vi "Demo_MakeData.vi"(11 "DataString":string) -> (2 "Data":u8[](array[numeric]), 3 "DataLen":u8)   [LabVIEW 2011]
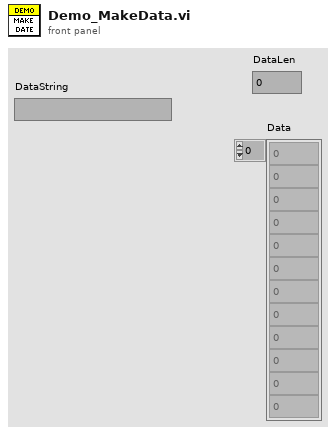
[diagram p1: front panel]
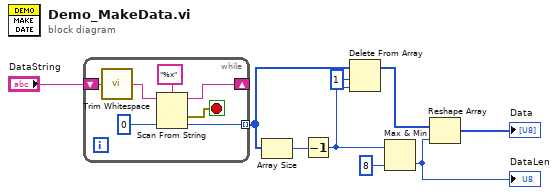
[diagram p0: block diagram]
diagram:
  n1 = while {
    shift-right: [w13] -> _
    shift-left: "DataString" -> [w16]
    tunnel: [w11] -> w8 mode=indexing
    stop <- w10 stop-if-true
    n2 = call <vilib>:"Trim Whitespace.vi"("string"=w16) -> ("trimmed string"=w15:string)  [unwired: 1 in]
    n3 = Scan From String(format string="%x" ("格式字符串"), input string=w15, default 1=u8 0) -> (remaining string=w13:string, error out=w10:errorcluster, output 1=w11:u8)  [unwired: 2 in, 1 out]
  }
  n4 = Array Size(array=w8) -> (size(s)=w6:i32)
  n5 = Decrement(x=w6) -> (x-1=w4:i32)
  n6 = Delete From Array(array=w8, length=1 ("长度"), index=w4) -> (array with subset deleted=w7:u8[])  [unwired: 1 out]
  n7 = Max & Min(x=w4, y=8 ("维数大小")) -> (min(x,y)=w1:i32)  [unwired: 1 out]
  "DataLen" <- w1
  n8 = Reshape Array(w7, w1) -> (→"Data":u8[])
